vi "Instrument Do Core.vi"(8 "error in (no error)":errorcluster, 9 "Instrument in":refnum<class "Instrument Driver.lvclass">, 10 "Actor in":refnum<class "Actor.lvclass">, 11 "DMM Config RTD Type Msg in":refnum<class "DMM Config RTD Type Msg.lvclass">) -> (0 "error out":errorcluster, 1 "Instrument out":refnum<class "Instrument Driver.lvclass">, 2 "Actor out":refnum<class "Actor.lvclass">, 3 "DMM Config RTD Type Msg out":refnum<class "DMM Config RTD Type Msg.lvclass">, 5 "Data":refnum<class "Data.lvclass">)   [LabVIEW 2020, in "DMM Msg.lvlib" / "DMM Config RTD Type Msg.lvclass"]
doc: "Set the RTD Type configuration on the DMM and return the Success boolean in a generic Boolean class."
uses:
  DMM Config RTD Type Msg.lvclass
  PPL/HDH.Actor Framework.Core.Actor.lvlibp/1abvi3w/vi.lib/ActorFramework/Actor/Actor.lvclass
  PPL/HDH.Data.Generic.lvlibp/Data.lvclass
  PPL/HDH.Actor Framework.Core.Instrument Driver.lvlibp/Instrument Driver/Instrument Driver.lvclass
  PPL/HDH.Driver.DMM.lvlibp/DMM Driver.lvclass
  C:/Current projects/WS/PPL/HDH.Actor Framework.Core.Instrument Driver.lvlibp/Instrument Driver/Instrument Driver.lvclass
  DMM Config RTD Type Msg.lvclass/DMM Config RTD Type Msg.ctl
  PPL/HDH.Data.Generic.lvlibp/Generic Data/Boolean/Boolean.lvclass
  C:/Current projects/WS/PPL/HDH.Data.Generic.lvlibp/Data.lvclass
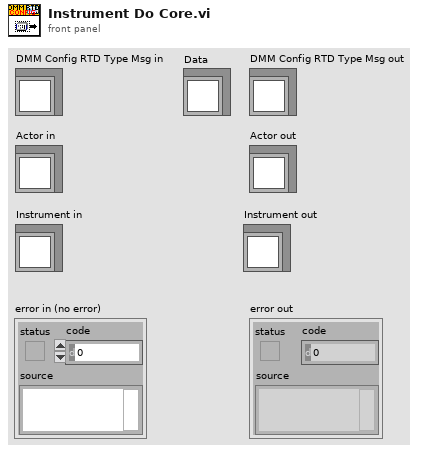
[diagram p1: front panel]
types:
  T1 = typedef "HDH.Driver.DMM.lvlibp/Ctl_RTDType.ctl" = enum16{"Custom", "Pt3750", "Pt3851", "Pt3911", "Pt3916", "Pt3920", "Pt3928"}
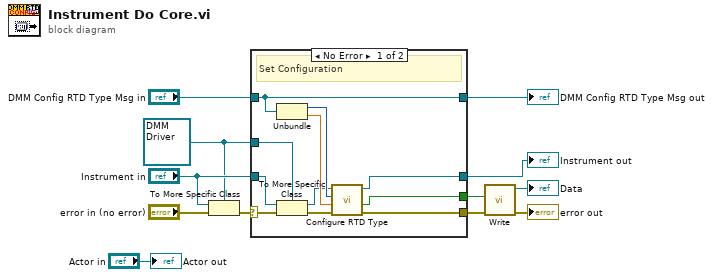
[diagram p0: block diagram]
diagram:
  w5 = refnum<class "DMM Driver.lvclass"> refnum ("HDH.Driver.DMM.lvlibp:DMM Driver.lvclass")
  n1 = To More Specific Class(target class=w5, reference="Instrument in", error in="error in (no error)") -> (error out=w10:errorcluster)  [unwired: 1 out]
  n2 = case shown="No Error" w10 {
    selector: w10 -> [w22 w25]
    tunnel: [w12 w25] -> w1
    tunnel: [w19 w24] -> w9
    tunnel: "DMM Config RTD Type Msg in" -> [w19 w24]
    tunnel: [w14 w23] -> w7
    tunnel: "Instrument in" -> [w21 w23]
    tunnel: w5 -> [w20 _]
    tunnel: [w18 _] -> w2
    frame No Error {
      # "Set Configuration"
      n3 = Unbundle(w19) -> (w17:T1, w16:dbl)
      n4 = To More Specific Class(target class=w20, reference=w21, error in=w22) -> (specific class reference=w15:refnum<class "DMM Driver.lvclass">, error out=w13:errorcluster)
      n5 = call-dynamic "Configure RTD Type.vi"("error in (no error)"=w13, "Resistance at 0°C(100Ohm)"=w16, "RTD Type"=w17, "DMM Driver in"=w15) -> ("error out"=w12:errorcluster, "Success?"=w18:bool, "DMM Driver out"=w14:refnum<class "DMM Driver.lvclass">)  [unwired: 5 in]
    }
    frame Error {
      # "Incorrect instrument - Return error"
    }
  }
  "error out" <- w1
  "DMM Config RTD Type Msg out" <- w9
  "Instrument out" <- w7
  n6 = call "Write.vi"("Boolean"=w2) -> ("Boolean out"=→"Data":refnum<class "Boolean.lvclass">)  [unwired: 10 in]
  "Actor out" <- "Actor in"
